vi "EncodeInLine.vi"(0 "Look Up Table":path, 1 "Final Sector Image Size":T4, 2 "Bypass Sector?":bool, 3 "Range Params":T2={"mb max"=-10.0, "mb min"=-60.0, "slope max"=4.0, "slope min"=-8.0, "int max"=5.0, "int min"=-85.0} {"int min" format="%.2f"; "int max" format="%.2f"; "slope min" format="%.2f"; "slope max" format="%.2f"; "mb min" format="%.2f"; "mb max" format="%.2f"}, 4 "Header In":T1={"header info"={"Header"="", "Head length"=0}, "A/D info"={"# rf points per line"=0, "# lines per scan"=0, "sample rate MHz"=0, "# A/D bits"=0, "# bytes per A/D"=0, "TGC Flag"=0, "A/D Type"=""}, "Tranducer Info"={"bandwidth"=0.0, "center freq"=0.0, "start freq"=0.0, "ID"=0}, "Scan Info"={"delay"=0.0, "pivot distance"=0.0, "sector scan angle"=0.0, "operator"="", "Scan Mode"="", "location"=""}, "Time/Date Info"={"date"="", "time"=""}, "RF Info"={"RF file name"="", "RF file att"="", "RF cal file name"="", "RF cal file att"=""}, "Patient Info"={"ID"="", "extended ID"="", "age"=0, "sex"="", "previously\nscanned"="", "PSA"=0.0, "LOS"=1, "Ethnicty 2"=3, "Race"=3}, "Tissue Type"={"organ"=0, "disease type"=0, "disease location"=0, "IQ_pts"=0, "RcvBuffer"=0, "RcvFrame"=0, "IQBuff"=0, "IQFrame"=0, "IQPage"=0}, "Votage scaling"={"Digitizer (dB)"=0.0, "Gain (dB)"=0.0, "Atten (dB)"=0.0}, "Comment"="", "Misc Info"={"avg num"=0, "c speed"=0, "Div By or SF zones"=0, "XMIT CHS"=0, "RCV CHS"=0, "Xmit angle"=0.0}, "Therapy Parameters"={"Theraputic Freq (MHz)"=0.1, "Time on (s)"=1.0, "Therapy amplitude (mV)"=50.0, "Lines Before"=20, "Lines After"=80}, "Scan Settings"={"Energy (uJ or V)"=0, "Damp (Ohm) or Fc"=0, "HP Filt (KHz)"=0, "LP Filt (MHz)"=0, "Gain (db)"=0, "prf (kHz)"=0.0, "Distance between\nscan lines (um)"=0, "Distance between\nscan planes (um)"=0, "Scan line gap (um)"=0.0, "Scan plane gap (um)"=0.0}, "Compression Parameters"={"F1 (MHz)"=0.0, "F2 (MHz)"=0.0, "% taper"=0.0, "duration"=0.0}, "Patient Info Xtra"={"First Name"="", "Last Name"="", "Notes"=""}, "ROI Box"=[]} {"Compression Parameters"."% taper" min=50 max=1000 format="%.2f"; "Compression Parameters"."F2 (MHz)" format="%.3f"; "Compression Parameters"."F1 (MHz)" format="%.3f"; "Scan Settings"."prf (kHz)" format="%.2f"; "Therapy Parameters"."Therapy amplitude (mV)" min=50 max=1000 format="%.2f"; "Therapy Parameters"."Time on (s)" format="%.3f"; "Therapy Parameters"."Theraputic Freq (MHz)" format="%.3f"; "Patient Info"."Race" items=["Am Ind or Alaska", "Asian", "Hawaiian, Pac Isl", "Black or Afr Amer", "White", "more than one race", "unknown"]; "Patient Info"."Ethnicty 2" items=["Hispanic", "Non-Hispanic", "unknown"]; "Patient Info"."LOS" items=["1", "2", "3", "4", "5"]; "Patient Info"."PSA" format="%.1f"; "Scan Info"."delay" format="%.2f"; "Scan Info"."pivot distance" format="%.2f"; "Scan Info"."sector scan angle" format="%.2f"; "Tranducer Info"."bandwidth" format="%.2f"; "Tranducer Info"."center freq" format="%.2f"; "Tranducer Info"."start freq" format="%.2f"}, 6 "PSA Value":dbl, 7 "intercept":dbl[][](array[numeric]), 8 "thresholds":T3={"T1"=5.0, "T2"=6.0, "T3"=6.5, "T4"=7.0, "T5"=8.0} {"T5" format="%.2f"; "T4" format="%.2f"; "T3" format="%.2f"; "T2" format="%.2f"; "T1" format="%.2f"}, 9 "midband fit":dbl[][](array[numeric])) -> (12 "Scale Score":dbl[][](array[numeric]), 14 "Score Sector image":dbl[][](array[numeric]), 15 "Colored MB":dbl[][](array[numeric]), 16 "colored Int":dbl[][](array[numeric]), 17 "Colored Score":dbl[][](array[numeric]), 19 "Range Params in LUT":T2={"mb max"=-20.0, "mb min"=-70.0, "slope max"=8.0, "slope min"=-8.0, "int max"=5.0, "int min"=-85.0} {"int min" format="%.2f"; "int max" format="%.2f"; "slope min" format="%.2f"; "slope max" format="%.2f"; "mb min" format="%.2f"; "mb max" format="%.2f"})   [LabVIEW 2022 SP3]
uses:
  ViewData/-ReadEye/Header.ctl
  <vilib>/Analysis/NI_AALBase.lvlib
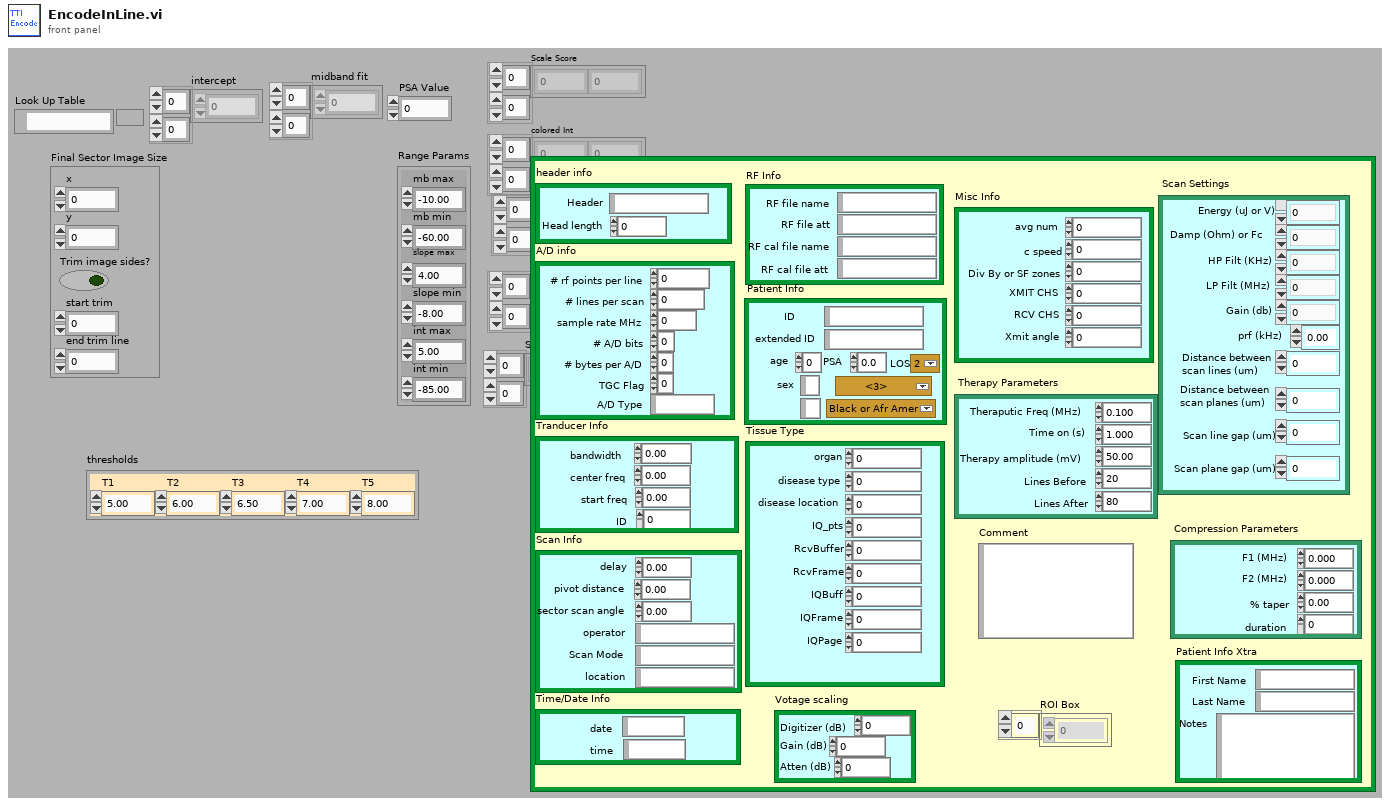
[diagram p1: front panel]
types:
  T1 = typedef "Header.ctl" = cluster{"header info":cluster{"Header":string, "Head length":i16}, "A/D info":cluster{"# rf points per line":u16, "# lines per scan":u16, "sample rate MHz":u16, "# A/D bits":i16, "# bytes per A/D":u16, "TGC Flag":u16, "A/D Type":string}, "Tranducer Info":cluster{"bandwidth":sgl, "center freq":sgl, "start freq":sgl, "ID":i32}, "Scan Info":cluster{"delay":sgl, "pivot distance":sgl, "sector scan angle":sgl, "operator":string, "Scan Mode":string, "location":string}, "Time/Date Info":cluster{"date":string, "time":string}, "RF Info":cluster{"RF file name":string, "RF file att":string, "RF cal file name":string, "RF cal file att":string}, "Patient Info":cluster{"ID":string, "extended ID":string, "age":u16, "sex":string, "previously\nscanned":string, "PSA":sgl, "LOS":u8, "Ethnicty 2":u8, "Race":u8}, "Tissue Type":cluster{"organ":i16, "disease type":i16, "disease location":i16, "IQ_pts":u16, "RcvBuffer":u8, "RcvFrame":u16, "IQBuff":u8, "IQFrame":u16, "IQPage":u8}, "Votage scaling":cluster{"Digitizer (dB)":sgl, "Gain (dB)":sgl, "Atten (dB)":sgl}, "Comment":string, "Misc Info":cluster{"avg num":u16, "c speed":i16, "Div By or SF zones":i16, "XMIT CHS":u8, "RCV CHS":u8, "Xmit angle":sgl}, "Therapy Parameters":cluster{"Theraputic Freq (MHz)":sgl, "Time on (s)":sgl, "Therapy amplitude (mV)":sgl, "Lines Before":u16, "Lines After":u16}, "Scan Settings":cluster{"Energy (uJ or V)":u8, "Damp (Ohm) or Fc":u8, "HP Filt (KHz)":u8, "LP Filt (MHz)":u8, "Gain (db)":u8, "prf (kHz)":sgl, "Distance between\nscan lines (um)":u16, "Distance between\nscan planes (um)":u16, "Scan line gap (um)":sgl, "Scan plane gap (um)":sgl}, "Compression Parameters":cluster{"F1 (MHz)":sgl, "F2 (MHz)":sgl, "% taper":sgl, "duration":sgl}, "Patient Info Xtra":cluster{"First Name":string, "Last Name":string, "Notes":string}, "ROI Box":u16[]}
  T2 = cluster{"mb max":dbl, "mb min":dbl, "slope max":dbl, "slope min":dbl, "int max":dbl, "int min":dbl}
  T3 = cluster{"T1":dbl, "T2":dbl, "T3":dbl, "T4":dbl, "T5":dbl}
  T4 = cluster{"x":i32, "y":i32, "Trim image sides?":bool, "start trim":i32, "end trim line":i32}
  T5 = cluster{"delay":sgl, "pivot distance":sgl, "sector scan angle":sgl, "operator":string, "Scan Mode":string, "location":string}
  T6 = cluster{"# rf points per line":u16, "# lines per scan":u16, "sample rate MHz":u16, "# A/D bits":i16, "# bytes per A/D":u16, "TGC Flag":u16, "A/D Type":string}
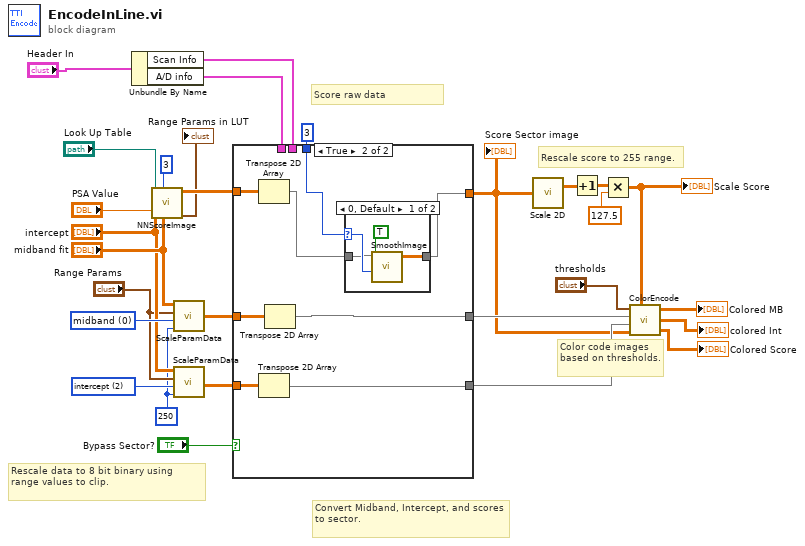
[diagram p0: block diagram]
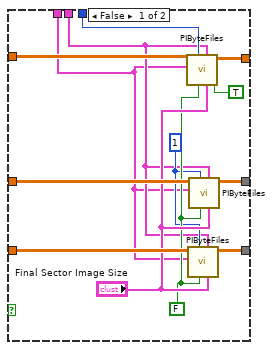
[diagram p2: hidden frame]
diagram:
  w24 = 250
  w25 = u16 2 items=["midband", "slope", "intercept"] ("parameter")
  w28 = u16 0 items=["midband", "slope", "intercept"] ("parameter")
  # "Color code images based on thresholds."
  # "Rescale score to 255 range."
  # "Convert Midband, Intercept, and scores to sector."
  # "Rescale data to 8 bit binary using range values to clip."
  # "Score raw data"
  n1 = Unbundle By Name("Header In") -> ("Scan Info"=w2:T5, "A/D info"=w1:T6)
  n2 = call "NNScoreImage.vi"("lookup path"="Look Up Table", "Window Av Size"=i8 3, "psa"="PSA Value", "Intercept"="intercept", "MidBand"="midband fit") -> ("score"=w6:dbl[][], "Range Params in LUT"=→"Range Params in LUT":T2)  [unwired: 4 out]
  n3 = call "ScaleParamData.vi"("max scale value"=w24, "parameter"=w28, "Range Params"="Range Params", "raw image data in"="midband fit") -> ("scaled output"=w16:dbl[][])
  n4 = call "ScaleParamData.vi"("max scale value"=w24, "parameter"=w25, "Range Params"="Range Params", "raw image data in"="intercept") -> ("scaled output"=w15:dbl[][])
  n5 = case shown="True" "Bypass Sector?" {
    tunnel: w16 -> [w42 w50]
    tunnel: w15 -> [w41 w49]
    tunnel: 3 -> [w39 w48]
    tunnel: [w37 w45] -> w13
    tunnel: [w36 w46] -> w12
    tunnel: [w35 w43] -> w9
    tunnel: w6 -> [w32 w47]
    tunnel: w2 -> [w31 _]
    tunnel: w1 -> [w30 _]
    frame False {
      w34 = 1
      w38 = FALSE
      n6 = call "PIByteFiles.vi"("use min z value?"=TRUE, "Final Sector Image Size"="Final Sector Image Size", "Scan Info"=w31, "Pre scale?"=w38, "Smooth factor"=w39, "A/D info"=w30, "raw image data in"=w32) -> ("raw sector out"=w35:dbl[][])  [unwired: 2 in, 2 out]
      n7 = call "PIByteFiles.vi"("Final Sector Image Size"="Final Sector Image Size", "Scan Info"=w31, "Pre scale?"=w38, "Smooth factor"=w34, "A/D info"=w30, "raw image data in"=w41) -> ("raw sector out"=w37:dbl[][])  [unwired: 3 in, 2 out]
      n8 = call "PIByteFiles.vi"("Final Sector Image Size"="Final Sector Image Size", "Scan Info"=w31, "Pre scale?"=w38, "Smooth factor"=w34, "A/D info"=w30, "raw image data in"=w42) -> ("raw sector out"=w36:dbl[][])  [unwired: 3 in, 2 out]
    }
    frame True {
      n9 = Transpose 2D Array(2D array=w47) -> (transposed array=w44:dbl[][])
      n10 = Transpose 2D Array(2D array=w49) -> (transposed array=w45:dbl[][])
      n11 = Transpose 2D Array(2D array=w50) -> (transposed array=w46:dbl[][])
      n12 = case shown="0, Default" w48 {
        selector: w48 -> [w52 _]
        tunnel: [w53 w55] -> w43
        tunnel: w44 -> [w51 w55]
        frame 0, Default {
          n13 = call "SmoothImage.vi"("sector array in"=w51, "Override min fill?"=TRUE, "Av size"=w52) -> ("Smoothed Sector w/Ave"=w53:cdb[][])  [unwired: 1 in, 3 out]
        }
        frame 1 {
        }
      }
    }
  }
  "Score Sector image" <- w9
  n14 = call <vilib>:"Scale 2D.vi"("X"=w9) -> ("Y=(X-offset)/scale"=w21:dbl[][])  [unwired: 3 out]
  n15 = Increment(x=w21) -> (x+1=w22:dbl[][])
  n16 = Multiply(x=w22, y=127.5) -> (x*y=w7:dbl[][])
  "Scale Score" <- w7
  n17 = call "ColorEncode.vi"("thresholds"="thresholds", "midband in"=w12, "intercept in"=w13, "score in"=w9, "scaled score"=w7) -> ("midband out"=→"Colored MB":dbl[][], "intercept out"=→"colored Int":dbl[][], "scaled score out"=→"Colored Score":dbl[][])
